vi "Add Frames and Signals.vi"(7 "Add Info?":bool, 8 "error in":errorcluster, 10 "Frames":T1[](array[typedef]), 11 "Parent Ref in":T2 format="%.0x") -> (0 "error out":errorcluster, 3 "XNET Signal Names":refnum<k21>[](array[refnum]))   [LabVIEW 2023, in "J1939 System Definition API Support.lvlib"]
uses:
  J1939 System Definition API Support.lvlib
  <vilib>/NI VeriStand/Custom Device API/Custom Device Item Ref.ctl
  Types/Add Item - Frame Cluster.ctl
  <vilib>/NI VeriStand/Custom Device API/Custom Device Channel.ctl
  <vilib>/NI VeriStand/Custom Device API/Custom Device Channel Type.ctl
  Addon/Addon Shared/Types/SPN Properties.ctl
  Addon/Addon Shared/SubVIs/Constants.vi
  <vilib>/NI/NI VeriStand Advanced SysDef API/_SubVIs/SysDef.Property.Set.U32.vi
  <resource>/objmgr/xnet.rc
  <vilib>/NI VeriStand/Custom Device API/Custom Device API.lvlib
  Addon/Addon Shared/J1939 Addon Shared.lvlib
  <vilib>/NI/NI VeriStand Advanced SysDef API/SysDef API/Advanced System Definition.lvlib
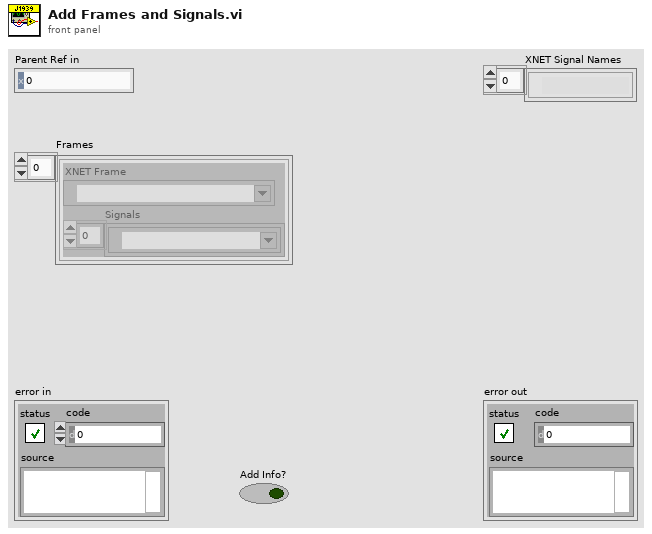
[diagram p1: front panel]
types:
  T1 = typedef "J1939 System Definition API Support.lvlib/Add Item - Frame Cluster.ctl" = cluster{"XNET Frame":refnum<k21>, "Signals":refnum<k21>[]}
  T2 = typedef "Custom Device API.lvlib/Custom Device Item Ref.ctl" = u64
  T3 = typedef "Custom Device API.lvlib/Custom Device Channel.ctl" = cluster{"Type":T4, "Units":string, "Default Value":dbl, "Faultable":bool, "Scalable":bool}
  T4 = typedef "Custom Device API.lvlib/Custom Device Channel Type.ctl" = enum16{"Input", "Output"}
  T5 = typedef "J1939 Addon Shared.lvlib/SPN Properties.ctl" = cluster{"Bytes":u32, "ScaleFac":dbl, "ScaleOff":dbl}
  T6 = typedef "Advanced System Definition.lvlib/TreeItem.Info.ctl" = cluster{"Name":string, "Description":string, "GUID":string, "Is Channel":bool, "Channel":T3, "Is Waveform":bool, "Waveform":T7}
  T7 = typedef "Custom Device API.lvlib/Custom Device Waveform.ctl" = cluster{"Data Type":T8, "Units":string}
  T8 = typedef "Custom Device API.lvlib/Custom Device Waveform DataType.ctl" = enum16{"Double", "Complex Double"}
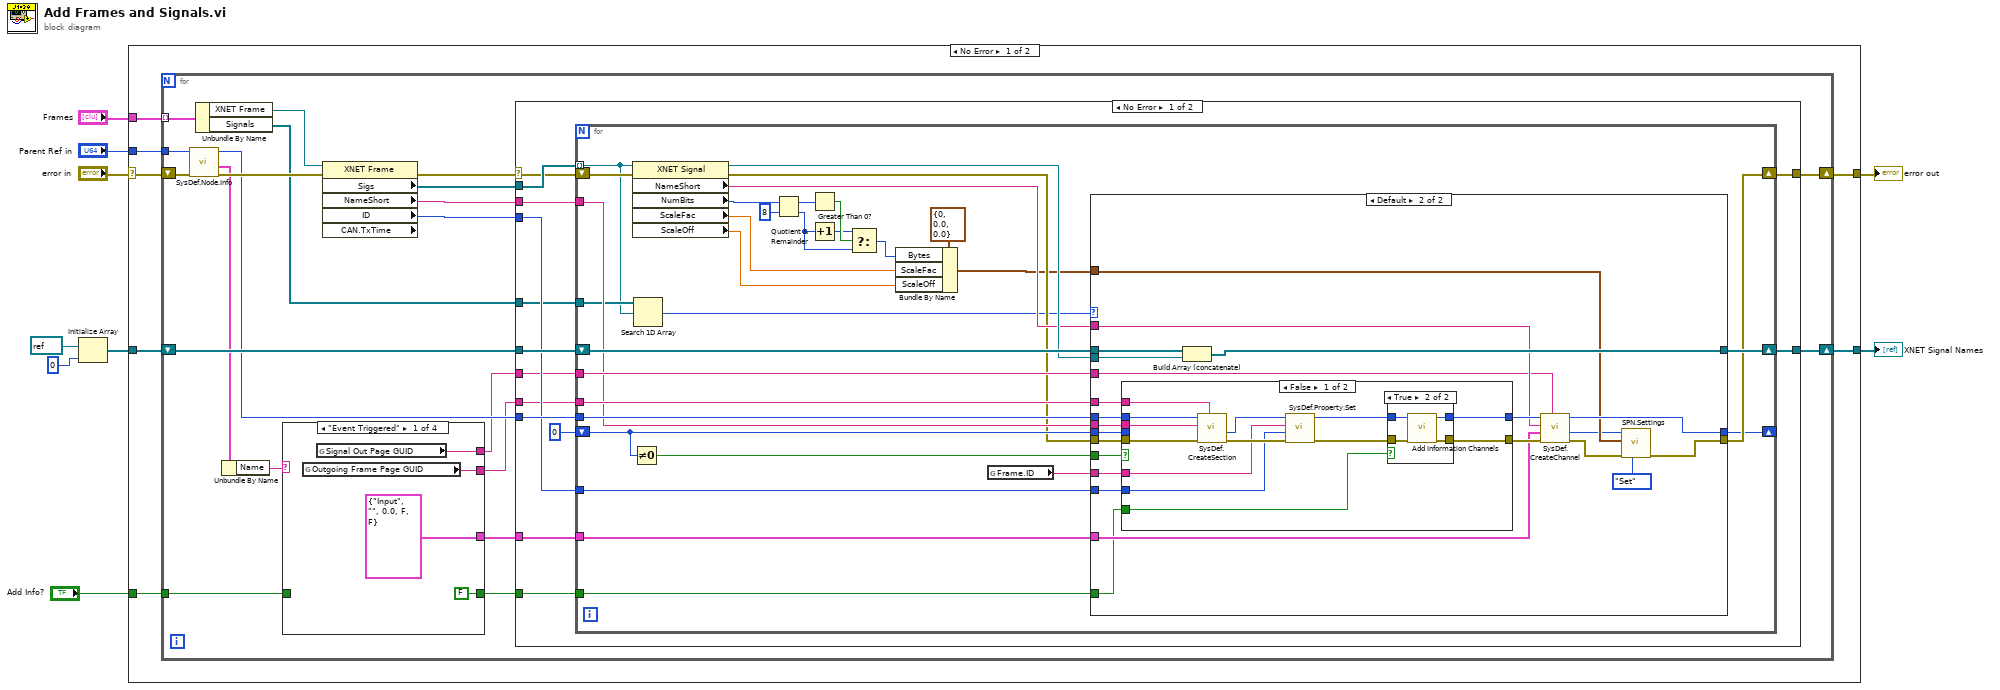
[diagram p0: block diagram]
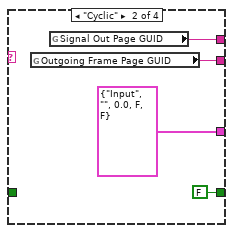
[diagram p2: hidden frame]
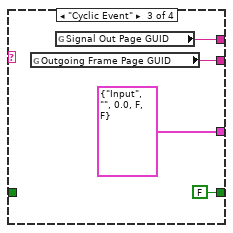
[diagram p3: hidden frame]
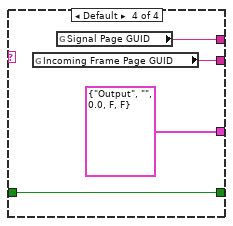
[diagram p4: hidden frame]
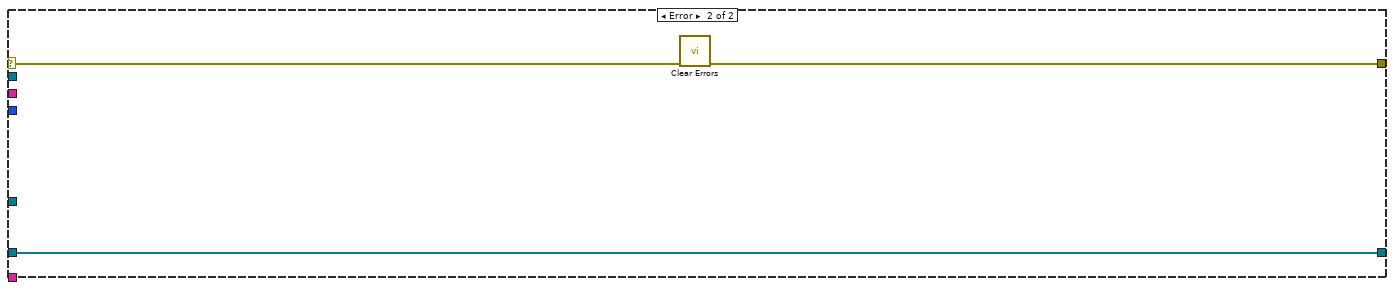
[diagram p8: hidden frame]
diagram:
  n1 = Initialize Array(refnum<k21> refnum ("XNET Signal"), 0 ("dimension size")) -> (w5:refnum<k21>[])
  n2 = case shown="No Error" "error in" {
    selector: "error in" -> [w14 w150]
    tunnel: [w16 w150] -> w9
    tunnel: "Frames" -> [w15 _]
    tunnel: [w13 _] -> w7
    tunnel: w5 -> [w12 _]
    tunnel: "Parent Ref in" -> [w11 _]
    tunnel: "Add Info?" -> [w10 _]
    frame No Error {
      n3 = for {
        shift-right: [w36] -> w16
        shift-left: w14 -> [w32]
        tunnel: w15 -> [w25] mode=indexing
        shift-right: [w34] -> w13
        shift-left: w12 -> [w35]
        tunnel: w11 -> [w30]
        tunnel: w10 -> [w18]
        n4 = call <vilib>:"SysDef.Node.Info.vi"("error in (no error)"=w32, "nodeID"=w30) -> ("error out"=w31:errorcluster, "Item Info"=w28:T6, "nodeID out"=w29:u64)  [unwired: 6 in, 1 out]
        n5 = Unbundle By Name(w25) -> ("XNET Frame"=w24:refnum<k21>, "Signals"=w23:refnum<k21>[])
        n6 = Unbundle By Name(w28) -> ("Name"=w22:string)
        n7 = case shown="\"Event Triggered\"" w22 {
          tunnel: [w40 w44 w48 w52] -> w20
          tunnel: [T3 {"Type"=enum."Input", "Units"="", "Default Value"=0.0, "Faultable"=FALSE, "Scalable"=FALSE} ("Channel") T3 {"Type"=enum."Input", "Units"="", "Default Value"=0.0, "Faultable"=FALSE, "Scalable"=FALSE} ("Channel") T3 {"Type"=enum."Input", "Units"="", "Default Value"=0.0, "Faultable"=FALSE, "Scalable"=FALSE} ("Channel") T3 {"Type"=enum."Output", "Units"="", "Default Value"=0.0, "Faultable"=FALSE, "Scalable"=FALSE} ("Channel")] -> w21
          tunnel: [w39 w43 w47 w51] -> w19
          tunnel: w18 -> [_ _ _ w50]
          tunnel: [FALSE ("Add Info?") FALSE ("Add Info?") FALSE ("Add Info?") w50] -> w17
          frame "Event Triggered" {
            n8 = global read "Constants.vi" "Outgoing Frame Page GUID"() -> (w40:string)
            n9 = global read "Constants.vi" "Signal Out Page GUID"() -> (w39:string)
          }
          frame "Cyclic" {
            n10 = global read "Constants.vi" "Outgoing Frame Page GUID"() -> (w44:string)
            n11 = global read "Constants.vi" "Signal Out Page GUID"() -> (w43:string)
          }
          frame "Cyclic Event" {
            n12 = global read "Constants.vi" "Outgoing Frame Page GUID"() -> (w48:string)
            n13 = global read "Constants.vi" "Signal Out Page GUID"() -> (w47:string)
          }
          frame Default {
            n14 = global read "Constants.vi" "Incoming Frame Page GUID"() -> (w52:string)
            n15 = global read "Constants.vi" "Signal Page GUID"() -> (w51:string)
          }
        }
        n16 = property class="XNET Frame" props=["Sigs", "NameShort", "ID", "CAN.TxTime"](reference=w24, error in=w31) -> (error out=w33:errorcluster, "Sigs"=w37:refnum<k21>[], "NameShort"=w27:string, "ID"=w26:u32)  [unwired: 2 out]
        n17 = case shown="No Error" w33 {
          selector: w33 -> [w60 w148]
          tunnel: w37 -> [w67 _]
          tunnel: w27 -> [w66 _]
          tunnel: [w65 w147] -> w36
          tunnel: w35 -> [w64 w149]
          tunnel: [w63 w149] -> w34
          tunnel: w29 -> [w62 _]
          tunnel: w26 -> [w59 _]
          tunnel: w19 -> [w58 _]
          tunnel: w20 -> [w57 _]
          tunnel: w21 -> [w56 _]
          tunnel: w23 -> [w55 _]
          tunnel: w17 -> [w54 _]
          frame No Error {
            n18 = for {
              tunnel: w67 -> [w81] mode=indexing
              tunnel: w66 -> [w84]
              shift-right: [w95] -> w65
              shift-left: w60 -> [w99]
              shift-right: [w98] -> w63
              shift-left: w64 -> [w97]
              tunnel: w62 -> [w94]
              shift-right: [w93] -> _
              shift-left: T2 0 ("Parent Ref out") -> [w92]
              tunnel: w59 -> [w89]
              tunnel: w58 -> [w87]
              tunnel: w57 -> [w86]
              tunnel: w56 -> [w85]
              tunnel: w55 -> [w82]
              tunnel: w54 -> [w68]
              n19 = Not Equal To 0?(x=w92) -> (x != 0?=w91:bool)
              n20 = property class="XNET Signal"(reference=w81, error in=w99) -> (reference out=w96:refnum<k21>, error out=w83:errorcluster, "NameShort"=w90:string, "NumBits"=w72:u32, "ScaleFac"=w71:dbl, "ScaleOff"=w70:dbl)
              n21 = Search 1D Array(1D array=w82, element=w81) -> (index of element=w80:i32)  [unwired: 1 in]
              n22 = Quotient & Remainder(x=w72, y=u32 8) -> (x-y*floor(x/y)=w78:u32, floor(x/y)=w76:u32)
              n23 = Greater Than 0?(x=w78) -> (x > 0?=w77:bool)
              n24 = Increment(x=w76) -> (x+1=w75:u32)
              n25 = Select(t=w75, s=w77, f=w76) -> (s? t:f=w74:u32)
              n26 = Bundle By Name(cluster=T5 {"Bytes"=0, "ScaleFac"=0.0, "ScaleOff"=0.0}, "Bytes"=w74, "ScaleFac"=w71, "ScaleOff"=w70) -> (w69:T5)
              n27 = global read "Constants.vi" "Frame.ID"() -> (w88:string)
              n28 = case shown="Default" w80 {
                tunnel: [w102 w123] -> w98
                tunnel: w97 -> [w102 w125]
                tunnel: w96 -> [_ w124]
                tunnel: w91 -> [_ w122]
                tunnel: w84 -> [_ w121]
                tunnel: w83 -> [w101 w120]
                tunnel: [w101 w104] -> w95
                tunnel: w94 -> [_ w119]
                tunnel: [w100 w116] -> w93
                tunnel: w92 -> [w100 w118]
                tunnel: w90 -> [_ w114]
                tunnel: w86 -> [_ w113]
                tunnel: w87 -> [_ w112]
                tunnel: w89 -> [_ w111]
                tunnel: w88 -> [_ w110]
                tunnel: w85 -> [_ w109]
                tunnel: w69 -> [_ w106]
                tunnel: w68 -> [_ w103]
                frame -1 {
                }
                frame Default {
                  n29 = case shown="False" w122 {
                    tunnel: w121 -> [w138 _]
                    tunnel: w120 -> [w137 w146]
                    tunnel: [w129 w146] -> w117
                    tunnel: w119 -> [w136 _]
                    tunnel: [w127 w145] -> w115
                    tunnel: w118 -> [_ w145]
                    tunnel: w113 -> [w135 _]
                    tunnel: w111 -> [w131 _]
                    tunnel: w110 -> [w132 _]
                    tunnel: w103 -> [w126 _]
                    frame False {
                      n30 = call <vilib>:"SysDef.CreateSection.vi"("GUID"=w135, "error in (no error)"=w137, "Name"=w138, "nodeID"=w136) -> ("error out"=w134:errorcluster, "New NodeID"=w133:u64)  [unwired: 4 in, 2 out]
                      n31 = call-poly <vilib>:"SysDef.Property.Set.vi"("error in (no error)"=w134, "Value"=w131, "Property Name"=w132, "nodeID"=w133) -> ("error out"=w130:errorcluster, "nodeID out"=w128:u64)  [unwired: 6 in]
                      n32 = case shown="True" w126 {
                        tunnel: w128 -> [w139 w144]
                        tunnel: [w139 w143] -> w127
                        tunnel: w130 -> [w140 w142]
                        tunnel: [w140 w141] -> w129
                        frame False {
                        }
                        frame True {
                          n33 = call "Add Information Channels.vi"("error in (no error)"=w142, "Node Ptr"=w144) -> ("error out"=w141:errorcluster, "Parent Ref out"=w143:T2)  [unwired: 8 in]
                        }
                      }
                    }
                    frame True {
                    }
                  }
                  n34 = Build Array (concatenate)(w125, w124) -> (w123:refnum<k21>[])
                  n35 = call <vilib>:"SysDef.CreateChannel.vi"("GUID"=w112, "error in (no error)"=w117, "Channel"=w109, "Name"=w114, "nodeID"=w115) -> ("error out"=w107:errorcluster, "New NodeID"=w105:u64, "nodeID out"=w116:u64)  [unwired: 3 in, 1 out]
                  n36 = call "SPN.Settings.vi"("Action"=enum8{"Get", "Set"}."Set", "error in (no error)"=w107, "SPN.Settings"=w106, "Item Ref in"=w105) -> ("error out"=w104:errorcluster)  [unwired: 5 in, 2 out]
                }
              }
            }
          }
          frame Error {
            n37 = call <vilib>:"Clear Errors.vi"("error in (no error)"=w148) -> ("error out"=w147:errorcluster)  [unwired: 5 in, 1 out]
          }
        }
      }
    }
    frame Error {
    }
  }
  "error out" <- w9
  "XNET Signal Names" <- w7
